vi "BPM_detektor(SUBVI).vi"(1 "Vzorkovacka":dbl, 2 "Vstupní signál":dbl[](array[numeric])) -> (0 "Hodnota BPM":dbl)   [LabVIEW 2025]
uses:
  <vilib>/Analysis/3filter.llb/Filter Passband Type.ctl
  <vilib>/Analysis/3filter.llb/Butterworth Filter (DBL).vi
  <vilib>/Analysis/NI_AALBase.lvlib
  <vilib>/Analysis/NI_AALPro.lvlib
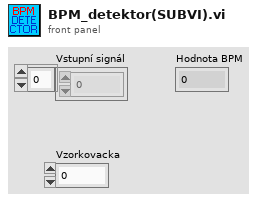
[diagram p1: front panel]
types:
  T1 = typedef "NI_AALBase.lvlib/Filter Passband Type.ctl" = enum32{"Lowpass", "Highpass", "Bandpass", "Bandstop"}
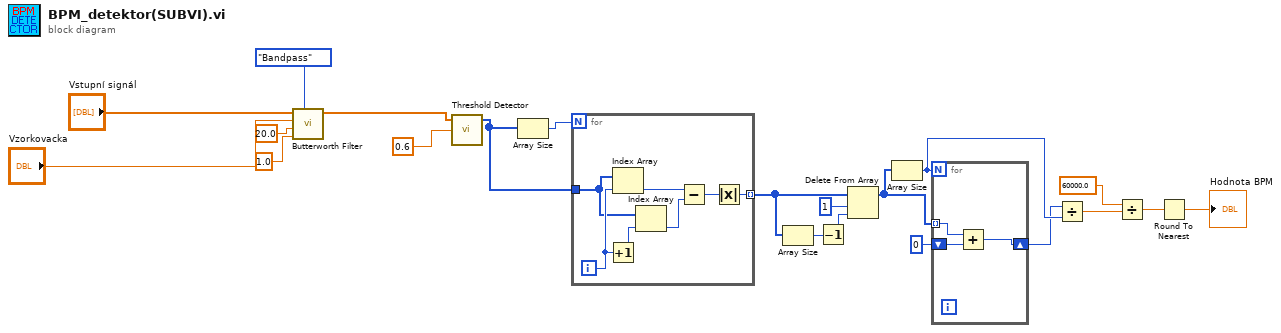
[diagram p0: block diagram]
diagram:
  n1 = call-poly <vilib>:"Butterworth Filter.vi"("filter type"=Filter_Passband_Type."Bandpass", "low cutoff freq: fl"=1.0, "high cutoff freq: fh"=20.0, "sampling freq: fs"="Vzorkovacka", "X"="Vstupní signál") -> ("Filtered X"=w7:dbl[])  [unwired: 3 in, 1 out]
  n2 = call <vilib>:"Threshold Detector.vi"("threshold"=0.6, "X"=w7) -> ("Indices"=w10:i32[])  [unwired: 1 in, 2 out]
  n3 = Array Size(array=w10) -> (size(s)=w9:i32)
  n4 = for {
    N: w9 -> [_]
    tunnel: w10 -> [w25]
    tunnel: [w22] -> w12 mode=indexing
    i -> [w27]
    n5 = Increment(x=w27) -> (x+1=w26:i32)
    n6 = Index Array(array=w25, index=w27) -> (element=w28:i32)
    n7 = Index Array(array=w25, index=w26) -> (element=w24:i32)
    n8 = Subtract(x=w28, y=w24) -> (x-y=w23:i32)
    n9 = Absolute Value(x=w23) -> (abs(x)=w22:i32)
  }
  n10 = Array Size(array=w12) -> (size(s)=w13:i32)
  n11 = Decrement(x=w13) -> (x-1=w14:i32)
  n12 = Delete From Array(array=w12, length=1, index=w14) -> (array with subset deleted=w15:i32[])  [unwired: 1 out]
  n13 = Array Size(array=w15) -> (size(s)=w18:i32)
  n14 = for {
    N: w18 -> [_]
    tunnel: w15 -> [w31] mode=indexing
    shift-right: [w30] -> w17
    shift-left: 0 -> [w29]
    n15 = Add(x=w31, y=w29) -> (x+y=w30:i32)
  }
  n16 = Divide(x=w17, y=w18) -> (x/y=w19:dbl)
  n17 = Divide(x=60000.0, y=w19) -> (x/y=w2:dbl)
  n18 = Round To Nearest(number=w2) -> (nearest integer value=→"Hodnota BPM":dbl)
